vi "frontPanel.vi"(8 "error in (no error)":errorcluster, 10 "ScriptEvent":refnum<class "ScriptEvent.lvclass">, 11 "ActionPanel in":refnum<class "RampAction.lvclass">) -> (0 "error out":errorcluster, 2 "ScriptEvent out":refnum<class "ScriptEvent.lvclass">, 3 "RampUpAction out":refnum<class "RampAction.lvclass">)   [LabVIEW 2011, in "Views.lvlib" / "ScriptEditor.lvlib" / "RampAction.lvclass"]
uses:
  RampAction.lvclass
  Tools/Scripting/ScriptingEvent/ScriptEvent.lvclass
  RampAction.lvclass/RampAction.ctl
  Tools/Scripting/ScriptingEvent/ScriptEvents/Ramp/RampEvent/RampEvent.lvclass
  ActionPanel.lvclass
panel:
  in  "Step Number":i32
  out "editing":bool
  in  "Value Step":dbl
  in  "States (End)":u16(ring)
  in  "Time Step":dbl format="%.6g"
  in  "End Value":string
  in  "Ramp Time":dbl format="%.6g"
  in  "States":u16(ring)
  out "ready?":bool
  in  "Dt":dbl format="%.6g"
  in  "Start Value":string
  in  "Start Time":dbl format="%.6g"
  in  "close":bool
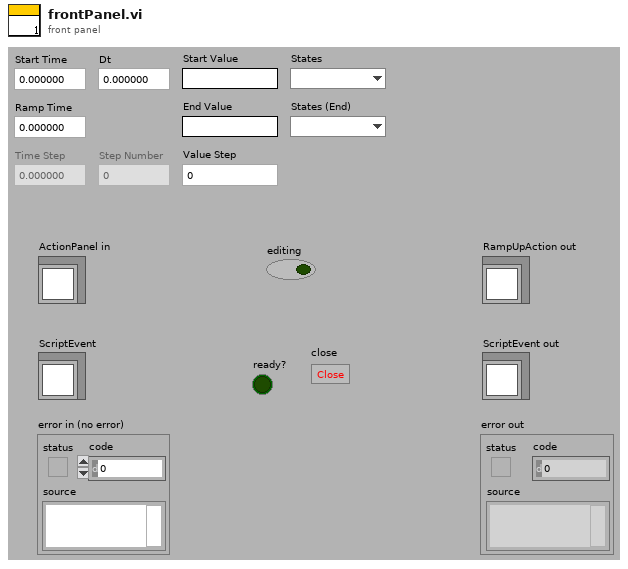
[diagram p1: front panel]
types:
  T1 = cluster{"Start Time":refnum<vi>, "Dt":refnum<vi>, "Start Value":refnum<vi>, "States":refnum<vi>, "Ramp Time":refnum<vi>, "Time Step":refnum<vi>, "End Value":refnum<vi>, "States (End)":refnum<vi>, "Value Step":refnum<vi>, "Step Number":refnum<vi>}
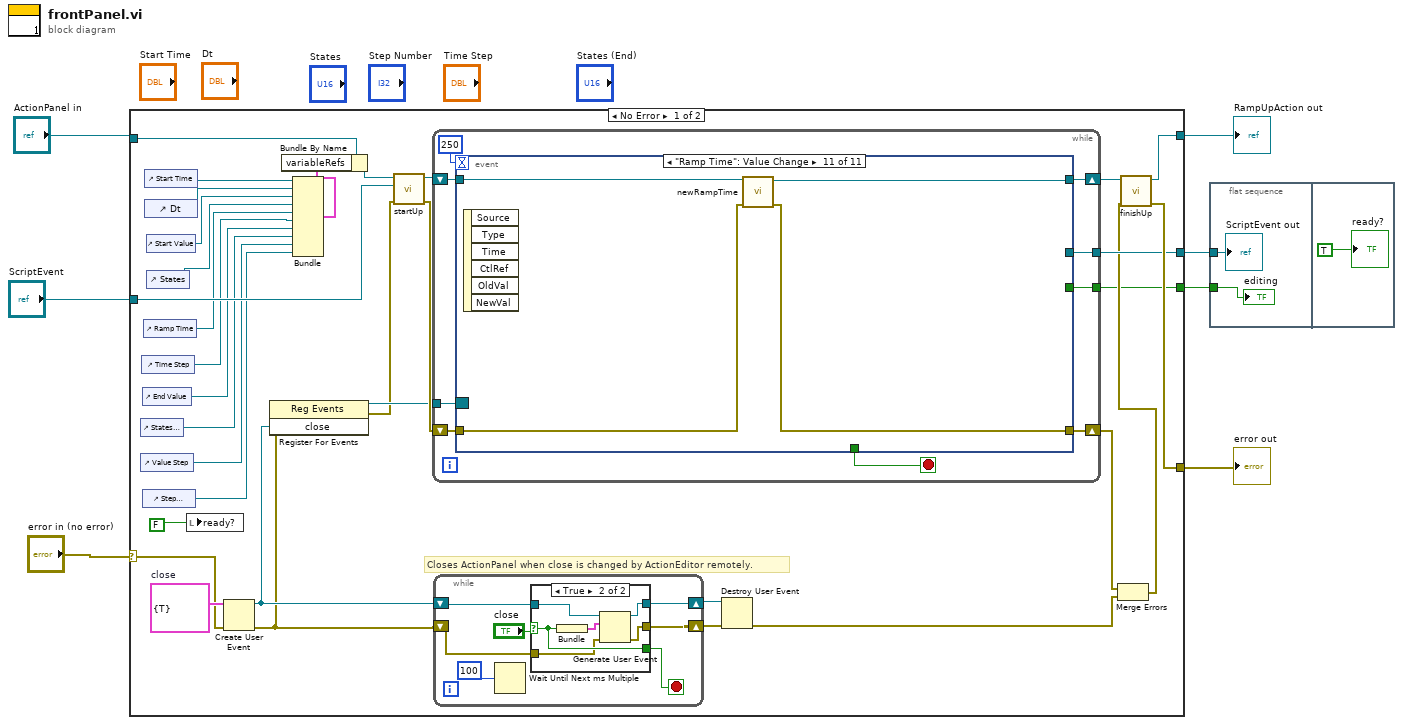
[diagram p0: block diagram]
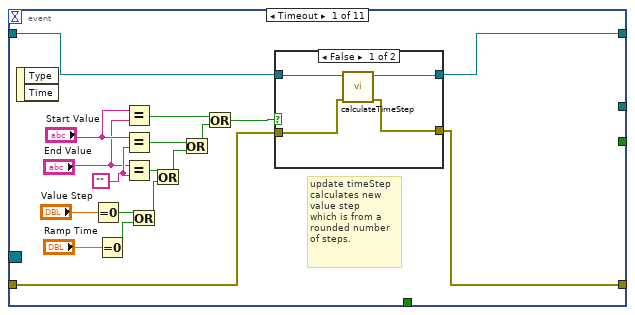
[diagram p3: hidden frame]
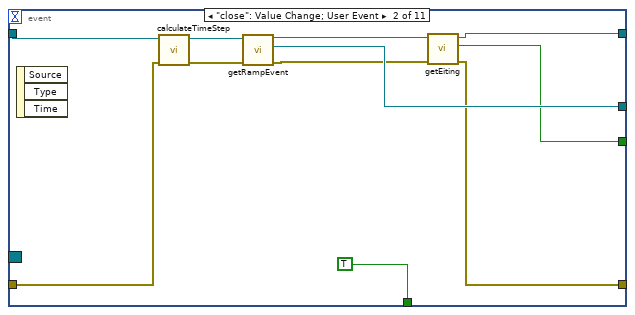
[diagram p5: hidden frame]
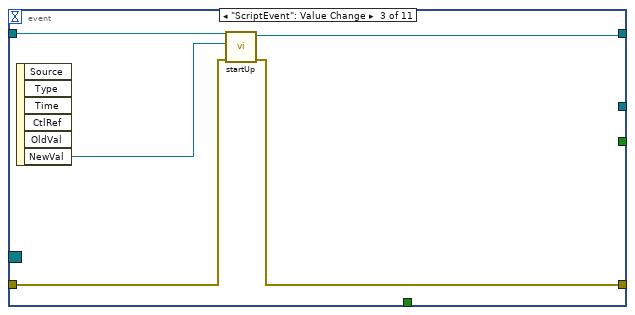
[diagram p6: hidden frame]
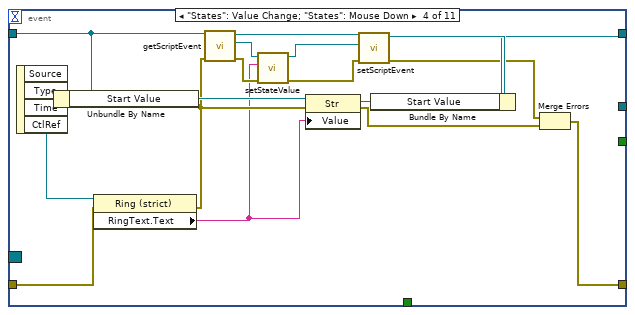
[diagram p7: hidden frame]
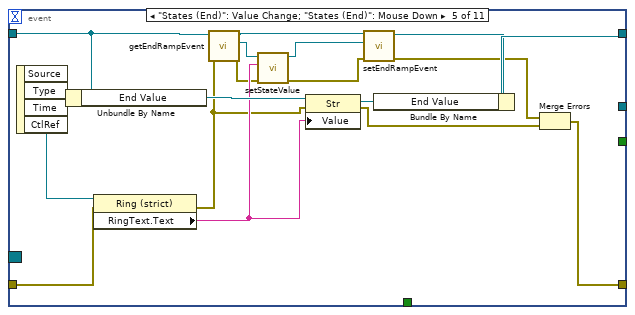
[diagram p8: hidden frame]
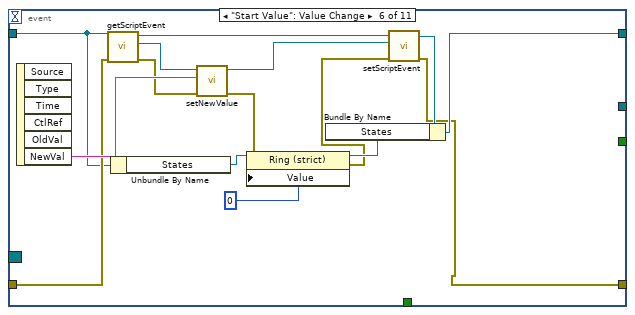
[diagram p9: hidden frame]
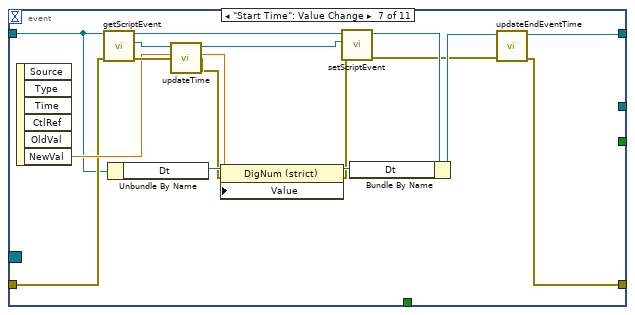
[diagram p10: hidden frame]
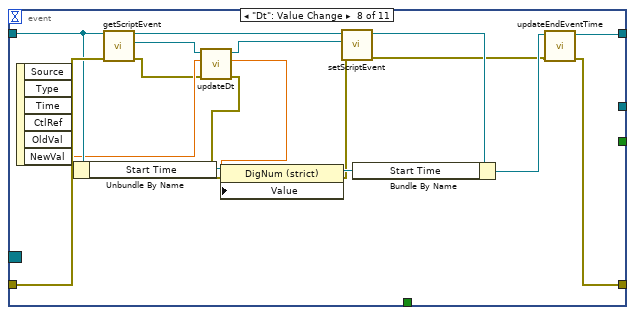
[diagram p11: hidden frame]
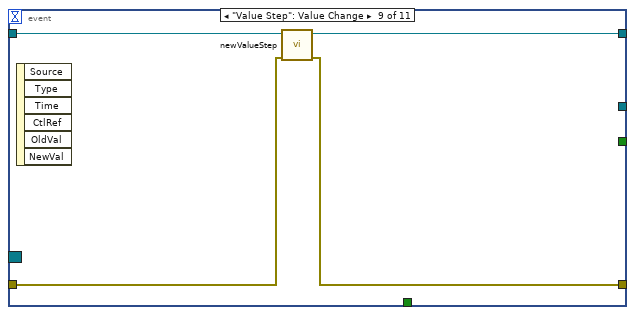
[diagram p12: hidden frame]
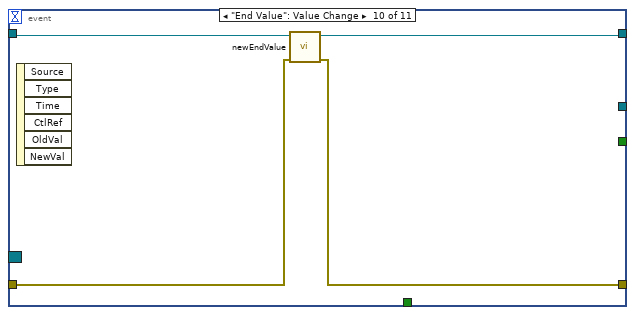
[diagram p13: hidden frame]
diagram:
  n1 = case shown="No Error" "error in (no error)" {
    selector: "error in (no error)" -> [w27 w201]
    tunnel: "ActionPanel in" -> [w9 w202]
    tunnel: [w32 w201] -> w3
    tunnel: [w33 w202] -> w5
    tunnel: "ScriptEvent" -> [w36 _]
    tunnel: [w30 _] -> w4
    tunnel: [w11 _] -> w1
    frame No Error {
      w28 = cluster{"close":bool} {"close"=TRUE}  # close
      # "Closes ActionPanel when close is changed by ActionEditor remotely."
      n2 = control-ref of="States (End)"() -> (w13:refnum<vi>)
      n3 = control-ref of="Value Step"() -> (w12:refnum<vi>)
      n4 = control-ref of="Time Step"() -> (w15:refnum<vi>)
      n5 = control-ref of="End Value"() -> (w14:refnum<vi>)
      n6 = control-ref of="Step Number"() -> (w10:refnum<vi>)
      n7 = control-ref of="Ramp Time"() -> (w16:refnum<vi>)
      n8 = control-ref of="Start Time"() -> (w39:refnum<vi>)
      n9 = control-ref of="Dt"() -> (w38:refnum<vi>)
      n10 = control-ref of="Start Value"() -> (w37:refnum<vi>)
      n11 = control-ref of="States"() -> (w29:refnum<vi>)
      n12 = local write "ready?"(FALSE) -> ()
      n13 = Create User Event(user event datatype=w28, error in=w27) -> (user event=w25:refnum<user-event>, error out=w22:errorcluster)
      n14 = register-events(error in=w22, w25) -> (reference out=w26:refnum<event-registration>, error out=w17:errorcluster)  [unwired: 1 in]
      n15 = Bundle("Start Time"=w39, "Dt"=w38, "Start Value"=w37, "States"=w29, "Ramp Time"=w16, "Time Step"=w15, "End Value"=w14, "States (End)"=w13, "Value Step"=w12, "Step Number"=w10) -> (w8:T1)  [unwired: 1 in]
      n16 = Bundle By Name(cluster=w9, "variableRefs"=w8) -> (w18:refnum<class "RampAction.lvclass">)
      n17 = call-dynamic "startUp.vi"("error in (no error)"=w17, "ScriptEvent"=w36, "RampAction in"=w18) -> ("error out"=w35:errorcluster, "RampAction out"=w40:refnum<class "RampAction.lvclass">)  [unwired: 7 in]
      n18 = while {
        shift-right: [w65] -> w34
        shift-left: w40 -> [w64]
        shift-right: [w62] -> w21
        shift-left: w35 -> [w63]
        tunnel: [w60] -> w30
        tunnel: w26 -> [w59]
        tunnel: [w57] -> w11
        stop <- w61 stop-if-true
        n19 = event shown="[10] \"Ramp Time\": Value Change" {
          selector: w59 -> [_ _ _ _ _ _ _ _ _ _ _]
          dyn-events: _ -> [_ _ _ _ _ _ _ _ _ _ _]
          timeout: 250 -> [_ _ _ _ _ _ _ _ _ _ _]
          tunnel: [w73 w95 w104 w111 w134 w144 w157 w174 w191 w195 w199] -> w65
          tunnel: w64 -> [w74 w92 w105 w117 w131 w149 w166 w186 w192 w196 w200]
          tunnel: [w71 w96 w101 w108 w132 w141 w155 w172 w189 w193 w197] -> w62
          tunnel: w63 -> [w72 w90 w102 w118 w138 w151 w167 w187 w190 w194 w198]
          tunnel: [_ TRUE _ _ _ _ _ _ _ _ _] -> w61
          tunnel: [_ w99 _ _ _ _ _ _ _ _ _] -> w60
          tunnel: [_ w94 _ _ _ _ _ _ _ _ _] -> w57
          event Timeout {
            w83 = ""
            # "update timeStep\ncalculates new\nvalue step\nwhich is from a \nrounded number\nof steps."
            n20 = event-data() -> ()  [unwired: 1 in, 2 out]
            n21 = Equal To 0?(x="Value Step") -> (x = 0?=w67:bool)
            n22 = Equal To 0?(x="Ramp Time") -> (x = 0?=w68:bool)
            n23 = Equal?(x="Start Value", y="End Value") -> (x = y?=w76:bool)
            n24 = Equal?(x="Start Value", y=w83) -> (x = y?=w81:bool)
            n25 = Equal?(x="End Value", y=w83) -> (x = y?=w80:bool)
            n26 = Or(x=w67, y=w68) -> (x .or. y?=w66:bool)
            n27 = Or(x=w80, y=w66) -> (x .or. y?=w75:bool)
            n28 = Or(x=w81, y=w75) -> (x .or. y?=w77:bool)
            n29 = Or(x=w76, y=w77) -> (x .or. y?=w70:bool)
            n30 = case shown="False" w70 {
              tunnel: w74 -> [w87 w89]
              tunnel: [w84 w89] -> w73
              tunnel: w72 -> [w86 w88]
              tunnel: [w85 w88] -> w71
              frame False {
                n31 = call "calculateTimeStep.vi"("error in (no error)"=w86, "RampAction in"=w87) -> ("error out"=w85:errorcluster, "RampAction out"=w84:refnum<class "RampAction.lvclass">)  [unwired: 8 in]
              }
              frame True {
              }
            }
          }
          event "close": Value Change; User Event {
            n32 = event-data() -> ()  [unwired: 1 in, 3 out]
            n33 = call "calculateTimeStep.vi"("error in (no error)"=w90, "RampAction in"=w92) -> ("error out"=w91:errorcluster, "RampAction out"=w93:refnum<class "RampAction.lvclass">)  [unwired: 8 in]
            n34 = call "getRampEvent.vi"("error in (no error)"=w91, "RampAction in"=w93) -> ("error out"=w97:errorcluster, "RampEvent"=w99:refnum<class "RampEvent.lvclass">, "RampAction out"=w98:refnum<class "RampAction.lvclass">)  [unwired: 7 in]
            n35 = call "getEiting.vi"("error in (no error)"=w97, "ActionPanel.lvclass in"=w98) -> ("error out"=w96:errorcluster, "editing?"=w94:bool, "ActionPanel.lvclass out"=w95:refnum<class "RampAction.lvclass">)  [unwired: 7 in]
          }
          event "ScriptEvent": Value Change {
            n36 = event-data() -> ("NewVal"=w103:refnum<class "ScriptEvent.lvclass">)  [unwired: 1 in, 5 out]
            n37 = call-dynamic "startUp.vi"("error in (no error)"=w102, "ScriptEvent"=w103, "RampAction in"=w105) -> ("error out"=w101:errorcluster, "RampAction out"=w104:refnum<class "RampAction.lvclass">)  [unwired: 7 in]
          }
          event "States": Value Change; "States": Mouse Down {
            n38 = event-data() -> ("CtlRef"=w119:refnum<vi>)  [unwired: 1 in, 3 out]
            n39 = Unbundle By Name(w117) -> ("Start Value"=w116:refnum<vi>)
            n40 = property class="Ring (strict)"(reference=w119, error in=w118) -> (error out=w115:errorcluster, "RingText.Text"=w114:string)  [unwired: 1 out]
            n41 = call "getScriptEvent.vi"("error in (no error)"=w115, "ActionPanel.lvclass in"=w117) -> ("error out"=w120:errorcluster, "ScriptEvent.lvclass"=w121:refnum<class "ScriptEvent.lvclass">, "ActionPanel.lvclass out"=w122:refnum<class "RampAction.lvclass">)  [unwired: 7 in]
            n42 = call "setStateValue.vi"("error in (no error)"=w120, "stateValue"=w114, "ScriptEvent in"=w121) -> ("error out"=w106:errorcluster, "ScriptEvent out"=w107:refnum<class "ScriptEvent.lvclass">)  [unwired: 7 in]
            n43 = property class="Str"(reference=w116, error in=w115, "Value"=w114) -> (reference out=w113:refnum<vi>, error out=w109:errorcluster)
            n44 = call "setScriptEvent.vi"("error in (no error)"=w106, "ScriptEvent.lvclass"=w107, "ActionPanel.lvclass in"=w122) -> ("error out"=w110:errorcluster, "ActionPanel.lvclass out"=w112:refnum<class "RampAction.lvclass">)  [unwired: 7 in]
            n45 = Bundle By Name(cluster=w112, "Start Value"=w113) -> (w111:refnum<class "RampAction.lvclass">)
            n46 = Merge Errors(w110, w109) -> (w108:errorcluster)
          }
          event "States (End)": Value Change; "States (End)": Mouse Down {
            n47 = event-data() -> ("CtlRef"=w139:refnum<vi>)  [unwired: 1 in, 3 out]
            n48 = Unbundle By Name(w131) -> ("End Value"=w137:refnum<vi>)
            n49 = property class="Ring (strict)"(reference=w139, error in=w138) -> (error out=w129:errorcluster, "RingText.Text"=w136:string)  [unwired: 1 out]
            n50 = call "getEndRampEvent.vi"("error in (no error)"=w129, "RampAction in"=w131) -> ("error out"=w125:errorcluster, "EndScriptEvent"=w130:refnum<class "ScriptEvent.lvclass">, "RampAction out"=w128:refnum<class "RampAction.lvclass">)  [unwired: 7 in]
            n51 = call "setStateValue.vi"("error in (no error)"=w125, "stateValue"=w136, "ScriptEvent in"=w130) -> ("error out"=w123:errorcluster, "ScriptEvent out"=w124:refnum<class "ScriptEvent.lvclass">)  [unwired: 7 in]
            n52 = property class="Str"(reference=w137, error in=w129, "Value"=w136) -> (reference out=w135:refnum<vi>, error out=w133:errorcluster)
            n53 = call "setEndRampEvent.vi"("error in (no error)"=w123, "EndScriptEvent"=w124, "RampAction in"=w128) -> ("error out"=w126:errorcluster, "RampAction out"=w127:refnum<class "RampAction.lvclass">)  [unwired: 7 in]
            n54 = Bundle By Name(cluster=w127, "End Value"=w135) -> (w134:refnum<class "RampAction.lvclass">)
            n55 = Merge Errors(w126, w133) -> (w132:errorcluster)
          }
          event "Start Value": Value Change {
            n56 = event-data() -> ("NewVal"=w152:string)  [unwired: 1 in, 5 out]
            n57 = call "getScriptEvent.vi"("error in (no error)"=w151, "ActionPanel.lvclass in"=w149) -> ("error out"=w150:errorcluster, "ScriptEvent.lvclass"=w153:refnum<class "ScriptEvent.lvclass">, "ActionPanel.lvclass out"=w154:refnum<class "RampAction.lvclass">)  [unwired: 7 in]
            n58 = Unbundle By Name(w149) -> ("States"=w148:refnum<vi>)
            n59 = call "setNewValue.vi"("error in (no error)"=w150, "newValue"=w152, "ScriptEvent.lvclass in"=w153) -> ("error out"=w143:errorcluster, "ScriptEvent.lvclass out"=w140:refnum<class "ScriptEvent.lvclass">)  [unwired: 7 in]
            n60 = property class="Ring (strict)"(reference=w148, error in=w143, "Value"=0) -> (reference out=w145:refnum<vi>, error out=w142:errorcluster)
            n61 = call "setScriptEvent.vi"("error in (no error)"=w142, "ScriptEvent.lvclass"=w140, "ActionPanel.lvclass in"=w154) -> ("error out"=w141:errorcluster, "ActionPanel.lvclass out"=w146:refnum<class "RampAction.lvclass">)  [unwired: 7 in]
            n62 = Bundle By Name(cluster=w146, "States"=w145) -> (w144:refnum<class "RampAction.lvclass">)
          }
          event "Start Time": Value Change {
            n63 = event-data() -> ("NewVal"=w168:dbl)  [unwired: 1 in, 5 out]
            n64 = call "getScriptEvent.vi"("error in (no error)"=w167, "ActionPanel.lvclass in"=w166) -> ("error out"=w169:errorcluster, "ScriptEvent.lvclass"=w170:refnum<class "ScriptEvent.lvclass">, "ActionPanel.lvclass out"=w171:refnum<class "RampAction.lvclass">)  [unwired: 7 in]
            n65 = Unbundle By Name(w166) -> ("Dt"=w165:refnum<vi>)
            n66 = call "updateTime.vi"("error in (no error)"=w169, "time"=w168, "ScriptEvent in"=w170) -> ("error out"=w164:errorcluster, "dt"=w163:dbl, "ScriptEvent out"=w159:refnum<class "ScriptEvent.lvclass">)  [unwired: 6 in]
            n67 = property class="DigNum (strict)"(reference=w165, error in=w164, "Value"=w163) -> (reference out=w162:refnum<vi>, error out=w160:errorcluster)
            n68 = call "setScriptEvent.vi"("error in (no error)"=w160, "ScriptEvent.lvclass"=w159, "ActionPanel.lvclass in"=w171) -> ("error out"=w156:errorcluster, "ActionPanel.lvclass out"=w161:refnum<class "RampAction.lvclass">)  [unwired: 7 in]
            n69 = Bundle By Name(cluster=w161, "Dt"=w162) -> (w158:refnum<class "RampAction.lvclass">)
            n70 = call "updateEndEventTime.vi"("error in (no error)"=w156, "RampAction in"=w158) -> ("error out"=w155:errorcluster, "RampAction out"=w157:refnum<class "RampAction.lvclass">)  [unwired: 8 in]
          }
          event "Dt": Value Change {
            n71 = event-data() -> ("NewVal"=w180:dbl)  [unwired: 1 in, 5 out]
            n72 = Unbundle By Name(w186) -> ("Start Time"=w185:refnum<vi>)
            n73 = call "getScriptEvent.vi"("error in (no error)"=w187, "ActionPanel.lvclass in"=w186) -> ("error out"=w179:errorcluster, "ScriptEvent.lvclass"=w181:refnum<class "ScriptEvent.lvclass">, "ActionPanel.lvclass out"=w188:refnum<class "RampAction.lvclass">)  [unwired: 7 in]
            n74 = call "updateDt.vi"("error in (no error)"=w179, "dt"=w180, "ScriptEvent in"=w181) -> ("error out"=w177:errorcluster, "time"=w178:dbl, "ScriptEvent out"=w176:refnum<class "ScriptEvent.lvclass">)  [unwired: 6 in]
            n75 = property class="DigNum (strict)"(reference=w185, error in=w177, "Value"=w178) -> (reference out=w184:refnum<vi>, error out=w182:errorcluster)
            n76 = call "setScriptEvent.vi"("error in (no error)"=w182, "ScriptEvent.lvclass"=w176, "ActionPanel.lvclass in"=w188) -> ("error out"=w173:errorcluster, "ActionPanel.lvclass out"=w183:refnum<class "RampAction.lvclass">)  [unwired: 7 in]
            n77 = Bundle By Name(cluster=w183, "Start Time"=w184) -> (w175:refnum<class "RampAction.lvclass">)
            n78 = call "updateEndEventTime.vi"("error in (no error)"=w173, "RampAction in"=w175) -> ("error out"=w172:errorcluster, "RampAction out"=w174:refnum<class "RampAction.lvclass">)  [unwired: 8 in]
          }
          event "Value Step": Value Change {
            n79 = event-data() -> ()  [unwired: 1 in, 6 out]
            n80 = call "newValueStep.vi"("error in (no error)"=w190, "RampAction in"=w192) -> ("error out"=w189:errorcluster, "RampAction out"=w191:refnum<class "RampAction.lvclass">)  [unwired: 8 in]
          }
          event "End Value": Value Change {
            n81 = event-data() -> ()  [unwired: 1 in, 6 out]
            n82 = call "newEndValue.vi"("error in (no error)"=w194, "RampAction in"=w196) -> ("error out"=w193:errorcluster, "RampAction out"=w195:refnum<class "RampAction.lvclass">)  [unwired: 8 in]
          }
          event "Ramp Time": Value Change {
            n83 = event-data() -> ()  [unwired: 1 in, 6 out]
            n84 = call "newRampTime.vi"("error in (no error)"=w198, "RampAction in"=w200) -> ("error out"=w197:errorcluster, "RampAction out"=w199:refnum<class "RampAction.lvclass">)  [unwired: 8 in]
          }
        }
      }
      n85 = while {
        shift-right: [w43] -> w23
        shift-left: w22 -> [w42]
        shift-right: [w44] -> w24
        shift-left: w25 -> [w47]
        stop <- w45 stop-if-true
        n86 = Wait Until Next ms Multiple(millisecond multiple=100) -> ()  [unwired: 1 out]
        n87 = case shown="True" "close" {
          selector: "close" -> [w50 w54]
          tunnel: w47 -> [w49 w56]
          tunnel: [w50 w54] -> w45
          tunnel: [w49 w53] -> w44
          tunnel: [w48 w52] -> w43
          tunnel: w42 -> [w48 w51]
          frame False {
          }
          frame True {
            n88 = Bundle(w54) -> (w55:cluster{bool})  [unwired: 1 in]
            n89 = Generate User Event(user event=w56, event data cluster=w55, error in=w51) -> (user event out=w53:refnum<user-event>, error out=w52:errorcluster)
          }
        }
      }
      n90 = Destroy User Event(user event=w24, error in=w23) -> (error out=w19:errorcluster)
      n91 = Merge Errors(w21, w19) -> (w20:errorcluster)
      n92 = call-dynamic "finishUp.vi"("error in (no error)"=w20, "RampAction in"=w34) -> ("error out"=w32:errorcluster, "RampAction out"=w33:refnum<class "RampAction.lvclass">)  [unwired: 8 in]
    }
    frame Error {
    }
  }
  "error out" <- w3
  "RampUpAction out" <- w5
  n93 = flat-sequence {
    tunnel: w4 -> [w204]
    tunnel: w1 -> [w203]
    frame #0 {
      "ScriptEvent out" <- w204
      "editing" <- w203
    }
    frame #1 {
      "ready?" <- TRUE
    }
  }
